vi "Write Reporting period.vi"(8 "error in (no error)":errorcluster, 10 "Reporting period":dbl, 11 "C37.118 Sim in":refnum<class "C37.118 Sim.lvclass">) -> (0 "error out":errorcluster, 3 "C37.118 Sim out":refnum<class "C37.118 Sim.lvclass">)   [LabVIEW 2014, in "SensorPlugins.lvlib" / "C37.118 Sim.lvclass"]
uses:
  C37.118 Sim.lvclass
  C37.118 Sim.lvclass/C37.118 Sim.ctl
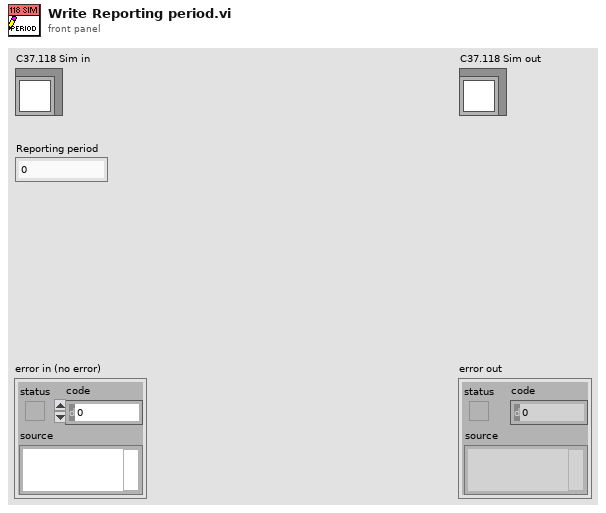
[diagram p1: front panel]
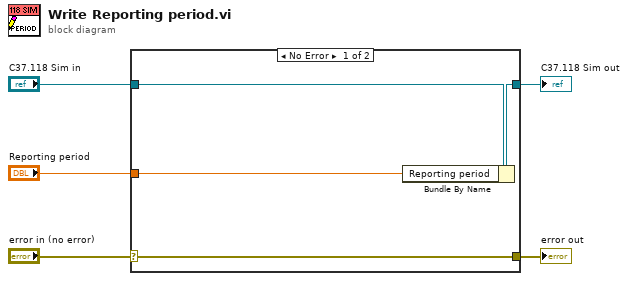
[diagram p0: block diagram]
diagram:
  n1 = case shown="No Error" "error in (no error)" {
    selector: "error in (no error)" -> [w9 w10]
    tunnel: [w9 w10] -> w4
    tunnel: [w7 w11] -> w2
    tunnel: "C37.118 Sim in" -> [w8 w11]
    tunnel: "Reporting period" -> [w6 _]
    frame No Error {
      n2 = Bundle By Name(cluster=w8, "Reporting period"=w6) -> (w7:refnum<class "C37.118 Sim.lvclass">)
    }
    frame Error {
    }
  }
  "error out" <- w4
  "C37.118 Sim out" <- w2
